vi "CreateWithReferencePackagePath.vi"(8 "Error In":errorcluster, 9 "Reference Package Version File (Optional)":path, 10 "Package Suffix":string="CE", 11 "Package Path":path) -> (0 "Error Out":errorcluster, 2 "Copy Exact Dependencies":string[](array[string]), 3 "Copy Exact Package Path":path)   [LabVIEW 2019, in "CEPM.lvlib"]
uses:
  CEPM.lvlib
  <vilib>/SLL Toolkit/SLL Table/_SubVIs/Get Table Data.vi
  <vilib>/SLL Toolkit/SLL File IO/Spreadsheet/SLL Spreadsheet.lvlib
  <vilib>/SLL Toolkit/SLL Table/SLL Table.lvclass
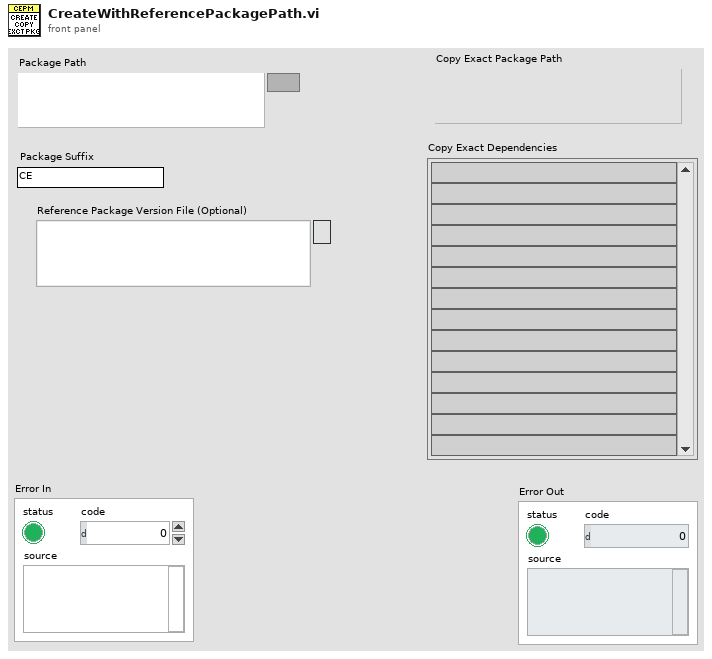
[diagram p1: front panel]
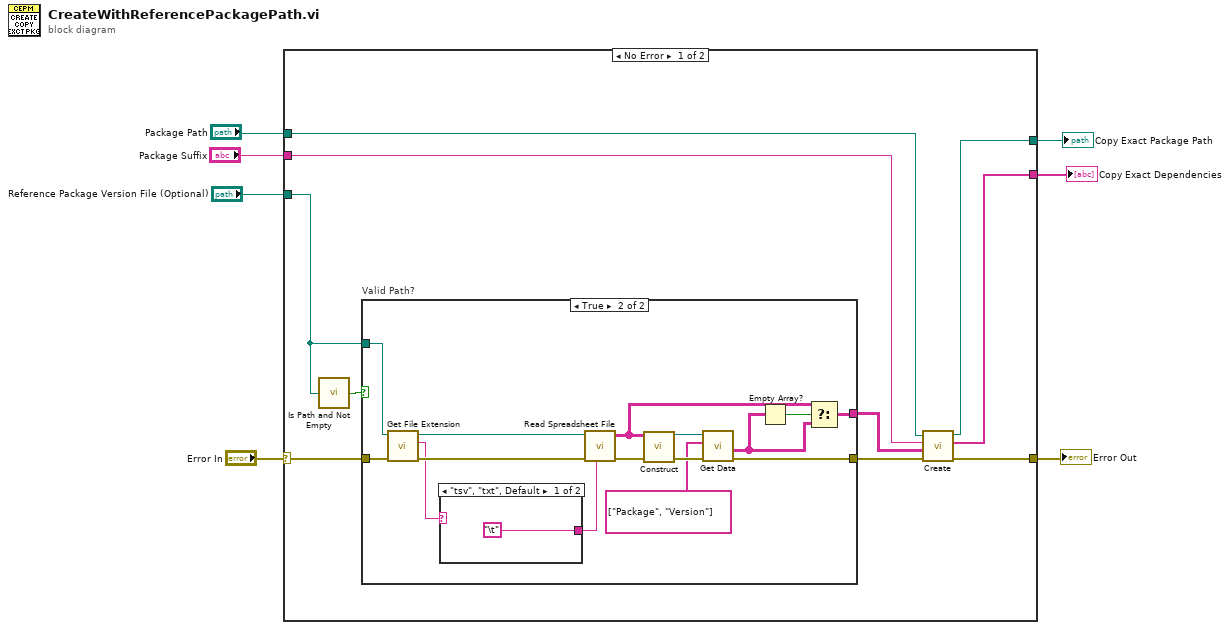
[diagram p0: block diagram]
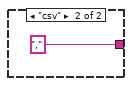
[diagram p3: hidden frame]
diagram:
  n1 = case shown="No Error" "Error In" {
    selector: "Error In" -> [w14 w36]
    tunnel: [w17 w36] -> w7
    tunnel: "Package Path" -> [w16 _]
    tunnel: "Package Suffix" -> [w15 _]
    tunnel: "Reference Package Version File (Optional)" -> [w12 _]
    tunnel: [w9 _] -> w2
    tunnel: [w8 _] -> w1
    frame No Error {
      n2 = call <vilib>:"Is Path and Not Empty.vi"("path"=w12) -> ("Is Path and Not Empty?"=w11:bool)  [unwired: 4 in]
      n3 = case "Valid Path?" shown="True" w11 {
        tunnel: [w18 w26] -> w13
        tunnel: [_ w19] -> w10
        tunnel: w12 -> [_ w31]
        tunnel: w14 -> [w18 w33]
        frame False {
        }
        frame True {
          n4 = call <vilib>:"Get File Extension.vi"("error in (no error)"=w33, "file"=w31) -> ("error out"=w32:errorcluster, "lowercase file extension"=w29:string, "dup file"=w30:path)  [unwired: 5 in, 2 out]
          n5 = case shown="\"tsv\", \"txt\", Default" w29 {
            tunnel: ["\t" "," ("Delimiter (tab)")] -> w28
            frame "tsv", "txt", Default {
            }
            frame "csv" {
            }
          }
          n6 = call <vilib>:"Read Spreadsheet File.vi"("Delimiter (tab)"=w28, "error in (no error)"=w32, "File Path"=w30) -> ("error out"=w27:errorcluster, "2D Array"=w21:string[][])  [unwired: 7 in]
          n7 = call <vilib>:"Construct.vi"("error in (no error)"=w27, "2D String with Headers"=w21) -> ("error out"=w25:errorcluster, "Table"=w24:refnum<class "SLL Table.lvclass">)  [unwired: 8 in]
          n8 = call-poly <vilib>:"Get Data.vi"("error in (no error)"=w25, "Header Order[] (Optional)"=string[] ["Package", "Version"], "SLL Table in"=w24) -> ("error out"=w26:errorcluster, "2D Data Out[][]"=w20:string[][])  [unwired: 5 in, 2 out]
          n9 = Empty Array?(array=w20) -> (empty?=w22:bool)
          n10 = Select(t=w21, s=w22, f=w20) -> (s? t:f=w19:string[][])
        }
      }
      n11 = call "Create.vi"("Error In"=w13, "Reference Package Versions (Optional)"=w10, "Package Suffix"=w15, "Package Path"=w16) -> ("Error Out"=w17:errorcluster, "Copy Exact Dependencies"=w8:string[], "Copy Exact Package Path"=w9:path)  [unwired: 5 in]
    }
    frame Error {
    }
  }
  "Error Out" <- w7
  "Copy Exact Package Path" <- w2
  "Copy Exact Dependencies" <- w1
